vi "S4GUI_003.vi"(7 "Tab ObsEng":enum32{"Obs", "CCD modes", "Guider", "Eng"}(tab)) -> ()   [LabVIEW 2018] (continued)
                    n884 = property on="Read Mode 2" class="Ring (strict)"("Blinking"=w1549) -> ()  [unwired: 2 in, 2 out]
                    n885 = property on="Pre-amplification Gain 2" class="Ring (strict)"("Blinking"=w1551) -> ()  [unwired: 2 in, 2 out]
                  }
                }
                n886 = local read "Cameras Cluster"() -> (w1515:T7)
                n887 = Bundle By Name(cluster=w1515, "Current Configuration.Image Initial Line 2"=w1478, "Current Configuration.Image Initial Column 2"=w1476, "Current Configuration.Image Final Line 2"=w1479, "Current Configuration.Image FInal Column 2"=w1477, "Current Configuration.Vertical Binning 2"=w1482, "Current Configuration.Horizontal Binning 2"=w1513, "Current Configuration.Pre-amplification Gain 2"=w1481, "Current Configuration.CCD EM Gain 2"=w1480, "Current Configuration.Readout Rate 2"=w1475, "Current Configuration.Shutter Openning Time 2"=w1512, "Current Configuration.Shutter Closing Time 2"=w1511, "Current Configuration.Vertical Shift Speed 2"=w1510, "Current Configuration.Read Mode 2"=w1509, "Current Configuration.Vertical Clock Voltage 2"=w1508, "Current Configuration.A/D Channel 2"=w1507, "Current Configuration.Shutter Mode 2"=w1504, "Current Configuration.Shutter TTL 2"=w1505, "Current Configuration.Trigger Mode 2"=w1483, "Current Configuration.Frame Transfer 2"=w1484, "Current Configuration.Acquisition Mode 2"=w1506, "Current Configuration.CCD EM Mode 2"=w1474) -> (w1514:T7)
                n888 = local write "PA2"(w1469) -> ()
                n889 = local write "B2"(w1468) -> ()
                n890 = local write "EA2"(w1470) -> ()
                n891 = local write "SI2"(w1465) -> ()
                n892 = local write "RO2"(w1466) -> ()
                n893 = local write "G2"(w1467) -> ()
                n894 = local write "Cameras Cluster"(w1514) -> ()
                n895 = Compound Arithmetic op=AND(w1489, w1488, w1487, w1486, w1462, w1461, w1485, w1496, w1495, w1494, w1493, w1492, w1491, w1490, w1503, w1502, w1501, w1500, w1499, w1498, w1497) -> (w1460:bool)
                "CCD checked 2" <- w1460
                n896 = disable-structure shown="Disabled" {
                  disable-tunnel: w1460 -> [w1517 _]
                  frame Disabled {
                    n897 = Select(t=u32 1244955, s=w1517, f=u32 16718848) -> (s? t:f=w1520:u32)
                    n898 = property on="CCD checked 2" class="Bool (strict)"("Caption.BG Color"=w1520) -> ()  [unwired: 2 in, 2 out]
                  }
                  frame Enabled {
                  }
                }
                n899 = property on="Acquisition Mode 2" class="Ring (strict)"("DisabledEnum"=w1463) -> ()  [unwired: 2 in, 2 out]
                n900 = property on="Readout Rate 2" class="Ring (strict)"("DisabledEnum"=w1463) -> ()  [unwired: 2 in, 2 out]
                n901 = property on="Vertical Shift Speed 2" class="Ring (strict)"("DisabledEnum"=w1463) -> ()  [unwired: 2 in, 2 out]
                n902 = property on="CCD EM Mode 2" class="Ring (strict)"("DisabledEnum"=w1463) -> ()  [unwired: 2 in, 2 out]
                n903 = property on="Shutter Openning Time 2" class="DigNum (strict)"("DisabledEnum"=w1463) -> ()  [unwired: 2 in, 2 out]
                n904 = property on="Shutter Closing Time 2" class="DigNum (strict)"("DisabledEnum"=w1463) -> ()  [unwired: 2 in, 2 out]
                n905 = property on="Vertical Binning 2" class="DigNum (strict)"("DisabledEnum"=w1463) -> ()  [unwired: 2 in, 2 out]
                n906 = property on="Horizontal Binning 2" class="DigNum (strict)"("DisabledEnum"=w1463) -> ()  [unwired: 2 in, 2 out]
                n907 = property on="Trigger Mode 2" class="Ring (strict)"("DisabledEnum"=w1463) -> ()  [unwired: 2 in, 2 out]
                n908 = property on="Read Mode 2" class="Ring (strict)"("DisabledEnum"=w1463) -> ()  [unwired: 2 in, 2 out]
                n909 = property on="Pre-amplification Gain 2" class="Ring (strict)"("DisabledEnum"=w1463) -> ()  [unwired: 2 in, 2 out]
                n910 = property on="CCD EM Gain 2" class="DigNum (strict)"("DisabledEnum"=w1463) -> ()  [unwired: 2 in, 2 out]
                n911 = property on="Shutter Mode 2" class="Ring (strict)"("DisabledEnum"=w1463) -> ()  [unwired: 2 in, 2 out]
                n912 = property on="Shutter TTL 2" class="Ring (strict)"("DisabledEnum"=w1463) -> ()  [unwired: 2 in, 2 out]
                n913 = property on="Image FInal Column 2" class="DigNum (strict)"("DisabledEnum"=w1463) -> ()  [unwired: 2 in, 2 out]
                n914 = property on="Frame Transfer 2" class="Bool (strict)"("DisabledEnum"=w1463) -> ()  [unwired: 2 in, 2 out]
                n915 = property on="Vertical Clock Voltage 2" class="Ring (strict)"("DisabledEnum"=w1463) -> ()  [unwired: 2 in, 2 out]
                n916 = property on="A/D Channel 2" class="DigNum (strict)"("DisabledEnum"=w1463) -> ()  [unwired: 2 in, 2 out]
                n917 = property on="Image Initial Line 2" class="DigNum (strict)"("DisabledEnum"=w1463) -> ()  [unwired: 2 in, 2 out]
                n918 = property on="Image Initial Column 2" class="DigNum (strict)"("DisabledEnum"=w1463) -> ()  [unwired: 2 in, 2 out]
                n919 = property on="Image Final Line 2" class="DigNum (strict)"("DisabledEnum"=w1463) -> ()  [unwired: 2 in, 2 out]
              }
              frame #17 {
                # "Carrega coluna do Channel 3"
                # "Aba:  Eng->Camera"
                n920 = Unbundle By Name(w1679) -> ("ChannelC_CCD"=w1649:T29, "CHC_Checked Params"=w1664:T14, "ChannelC_Status.connection"=w1642:bool)
                n921 = Unbundle By Name(w1664) -> ("ACQUISITION_MODE"=w1631:bool, "TRIGGER_MODE"=w1630:bool, "READ_MODE"=w1629:bool, "PREAMP"=w1628:bool, "READOUT_RATE"=w1627:bool, "VERTICAL_SHIFT_SPEED"=w1626:bool, "EM_MODE"=w1625:bool, "EM_GAIN"=w1662:bool, "SHUTTER_MODE"=w1661:bool, "SHUTTER_TTL"=w1660:bool, "SHUTTER_OPENING_TIME"=w1659:bool, "SHUTTER_CLOSING_TIME"=w1641:bool, "VBIN"=w1633:bool, "HBIN"=w1632:bool, "INITIAL_LINE"=w1640:bool, "INITIAL_COLUMN"=w1639:bool, "FINAL_LINE"=w1638:bool, "FINAL_COLUMN"=w1637:bool, "FRAME_TRANSFER"=w1636:bool, "VERTICAL_CLOCK_VOLTAGE"=w1635:bool, "AD_CHANNEL"=w1634:bool)
                n922 = case shown="True" w1642 {
                  tunnel: w1649 -> [_ w1732]
                  tunnel: [w1725 w1731] -> w1648
                  tunnel: [w1725 w1730] -> w1647
                  tunnel: [w1725 w1729] -> w1646
                  tunnel: [w1725 w1728] -> w1645
                  tunnel: [w1725 w1727] -> w1644
                  tunnel: [w1725 w1726] -> w1643
                  frame False {
                    w1725 = ""
                  }
                  frame True {
                    n923 = stacked-sequence "Atualizacao dos indicadores inferiores do CANAL C da tela principal" {
                      tunnel: w1732 -> [w1747 w1750 w1755 w1764 w1767 w1771]
                      tunnel: [w1733 _ _ _ _ _] -> w1731
                      tunnel: [_ w1748 _ _ _ _] -> w1730
                      tunnel: [_ _ w1753 _ _ _] -> w1729
                      tunnel: [_ _ _ w1758 _ _] -> w1728
                      tunnel: [_ _ _ _ w1765 _] -> w1727
                      tunnel: [_ _ _ _ _ w1768] -> w1726
                      frame #0 {
                        # "SubImage"
                        n924 = Unbundle By Name(w1747) -> ("INITIAL_LINE"=w1745:u16, "FINAL_LINE"=w1744:u16, "INITIAL_COLUMN"=w1743:u16, "FINAL_COLUMN"=w1742:u16)
                        n925 = Number To Decimal String(number=w1745) -> (decimal integer string=w1741:string)  [unwired: 1 in]
                        n926 = Number To Decimal String(number=w1744) -> (decimal integer string=w1739:string)  [unwired: 1 in]
                        n927 = Number To Decimal String(number=w1743) -> (decimal integer string=w1737:string)  [unwired: 1 in]
                        n928 = Number To Decimal String(number=w1742) -> (decimal integer string=w1735:string)  [unwired: 1 in]
                        n929 = Concatenate Strings("[", w1741, ":", w1739, ",", w1737, ":", w1735, "]") -> (w1733:string)
                      }
                      frame #1 {
                        # "Em Active"
                        n930 = Unbundle By Name(w1750) -> ("EM_MODE"=w1749:u8)
                        n931 = case shown="0, Default" w1749 {
                          tunnel: ["Electron M." ("EmActive1") "Convent." ("EmActive1")] -> w1748
                          frame 0, Default {
                          }
                          frame 1 {
                          }
                        }
                      }
                      frame #2 {
                        # "Pre Amp"
                        n932 = Unbundle By Name(w1755) -> ("PREAMP"=w1754:u8)
                        n933 = case shown="1" w1754 {
                          tunnel: ["Gain 1" ("EmActive1") "Gain 2" ("EmActive1")] -> w1753
                          frame 0, Default {
                          }
                          frame 1 {
                          }
                        }
                      }
                      frame #3 {
                        # "Binning"
                        n934 = Unbundle By Name(w1764) -> ("VBIN"=w1763:u16, "HBIN"=w1762:u16)
                        n935 = Number To Decimal String(number=w1762) -> (decimal integer string=w1759:string)  [unwired: 1 in]
                        n936 = Number To Decimal String(number=w1763) -> (decimal integer string=w1761:string)  [unwired: 1 in]
                        n937 = Concatenate Strings(w1761, "x", w1759) -> (w1758:string)
                      }
                      frame #4 {
                        # "Gain"
                        n938 = Unbundle By Name(w1767) -> ("EM_GAIN"=w1766:u16)
                        n939 = Number To Decimal String(number=w1766) -> (decimal integer string=w1765:string)  [unwired: 1 in]
                      }
                      frame #5 {
                        # "Readout"
                        n940 = Unbundle By Name(w1771) -> ("EM_MODE"=w1770:u8, "READOUT_RATE"=w1769:u8)
                        n941 = case shown="0, Default" w1770 {
                          tunnel: w1769 -> [w1773 w1779]
                          tunnel: [w1772 w1778] -> w1768
                          frame 0, Default {
                            n942 = case shown="3" w1773 {
                              tunnel: ["30 MHz" ("EmActive1") "20 MHz" ("EmActive1") "10 MHz" ("EmActive1") "1 MHz" ("EmActive1")] -> w1772
                              frame 0, Default {
                              }
                              frame 1 {
                              }
                              frame 2 {
                              }
                              frame 3 {
                              }
                            }
                          }
                          frame 1 {
                            n943 = case shown="1" w1779 {
                              tunnel: ["1 MHz" ("EmActive1") "0.1 MHz" ("EmActive1")] -> w1778
                              frame 0, Default {
                              }
                              frame 1 {
                              }
                            }
                          }
                        }
                      }
                    }
                  }
                }
                n944 = Unbundle By Name(w1649) -> ("INITIAL_LINE"=w1654:u16, "INITIAL_COLUMN"=w1652:u16, "FINAL_LINE"=w1655:u16, "FINAL_COLUMN"=w1653:u16, "VBIN"=w1658:u16, "HBIN"=w1676:u16, "PREAMP"=w1657:u8, "EM_GAIN"=w1656:u16, "READOUT_RATE"=w1651:u8, "SHUTTER_OPENNING_TIME"=w1675:u16, "SHUTTER_CLOSING_TIME"=w1674:u16, "VERTICAL_SHIFT_SPEED"=w1673:u8, "READ_MODE"=w1672:u8, "VERTICAL_CLOCK_VOLTAGE"=w1671:u8, "AD_CHANNEL"=w1670:u32, "SHUTTER_MODE"=w1665:u8, "SHUTTER_TTL"=w1666:u8, "TRIGGER_MODE"=w1667:u8, "FRAME_TRANSFER"=w1668:bool, "ACQUISITION_MODE"=w1669:u8, "EM_MODE"=w1650:u8)
                n945 = local read "CH3 on"() -> (w1624:bool)
                n946 = case shown="True" w1624 {
                  tunnel: w1662 -> [_ w1705]
                  tunnel: w1661 -> [_ w1704]
                  tunnel: w1660 -> [_ w1702]
                  tunnel: w1659 -> [_ w1701]
                  tunnel: w1641 -> [_ w1700]
                  tunnel: w1640 -> [_ w1699]
                  tunnel: w1639 -> [_ w1698]
                  tunnel: w1638 -> [_ w1697]
                  tunnel: w1637 -> [_ w1696]
                  tunnel: w1636 -> [_ w1695]
                  tunnel: w1635 -> [_ w1694]
                  tunnel: w1634 -> [_ w1693]
                  tunnel: w1633 -> [_ w1692]
                  tunnel: w1632 -> [_ w1691]
                  tunnel: w1631 -> [_ w1690]
                  tunnel: w1630 -> [_ w1689]
                  tunnel: w1629 -> [_ w1688]
                  tunnel: w1628 -> [_ w1687]
                  tunnel: w1627 -> [_ w1686]
                  tunnel: w1626 -> [_ w1685]
                  tunnel: w1625 -> [_ w1684]
                  tunnel: [T12."Disabled and Grayed Out" ("Disabled") T12."Enabled" ("Disabled")] -> w1623
                  frame False {
                    w1680 = FALSE
                    n947 = property on="Image Initial Line 3" class="DigNum (strict)"("Blinking"=w1680) -> ()  [unwired: 2 in, 2 out]
                    n948 = property on="Image Initial Column 3" class="DigNum (strict)"("Blinking"=w1680) -> ()  [unwired: 2 in, 2 out]
                    n949 = property on="Image Final Line 3" class="DigNum (strict)"("Blinking"=w1680) -> ()  [unwired: 2 in, 2 out]
                    n950 = property on="Image FInal Column 3" class="DigNum (strict)"("Blinking"=w1680) -> ()  [unwired: 2 in, 2 out]
                    n951 = property on="Frame Transfer 3" class="Bool (strict)"("Blinking"=w1680) -> ()  [unwired: 2 in, 2 out]
                    n952 = property on="Vertical Clock Voltage 3" class="Ring (strict)"("Blinking"=w1680) -> ()  [unwired: 2 in, 2 out]
                    n953 = property on="A/D Channel 3" class="DigNum (strict)"("Blinking"=w1680) -> ()  [unwired: 2 in, 2 out]
                    n954 = property on="CCD EM Gain 3" class="DigNum (strict)"("Blinking"=w1680) -> ()  [unwired: 2 in, 2 out]
                    n955 = property on="Shutter Mode 3" class="Ring (strict)"("Blinking"=w1680) -> ()  [unwired: 2 in, 2 out]
                    n956 = property on="Shutter TTL 3" class="Ring (strict)"("Blinking"=w1680) -> ()  [unwired: 2 in, 2 out]
                    n957 = property on="Shutter Openning Time 3" class="DigNum (strict)"("Blinking"=w1680) -> ()  [unwired: 2 in, 2 out]
                    n958 = property on="Shutter Closing Time 3" class="DigNum (strict)"("Blinking"=w1680) -> ()  [unwired: 2 in, 2 out]
                    n959 = property on="Vertical Binning 3" class="DigNum (strict)"("Blinking"=w1680) -> ()  [unwired: 2 in, 2 out]
                    n960 = property on="Horizontal Binning 3" class="DigNum (strict)"("Blinking"=w1680) -> ()  [unwired: 2 in, 2 out]
                    n961 = property on="Acquisition Mode 3" class="Ring (strict)"("Blinking"=w1680) -> ()  [unwired: 2 in, 2 out]
                    n962 = property on="Vertical Shift Speed 3" class="Ring (strict)"("Blinking"=w1680) -> ()  [unwired: 2 in, 2 out]
                    n963 = property on="Trigger Mode 3" class="Ring (strict)"("Blinking"=w1680) -> ()  [unwired: 2 in, 2 out]
                    n964 = property on="Read Mode 3" class="Ring (strict)"("Blinking"=w1680) -> ()  [unwired: 2 in, 2 out]
                    n965 = property on="Readout Rate 3" class="Ring (strict)"("Blinking"=w1680) -> ()  [unwired: 2 in, 2 out]
                    n966 = property on="CCD EM Mode 3" class="Ring (strict)"("Blinking"=w1680) -> ()  [unwired: 2 in, 2 out]
                    n967 = property on="Pre-amplification Gain 3" class="Ring (strict)"("Blinking"=w1680) -> ()  [unwired: 2 in, 2 out]
                  }
                  frame True {
                    n968 = Not(x=w1699) -> (.not. x?=w1682:bool)
                    n969 = Not(x=w1698) -> (.not. x?=w1723:bool)
                    n970 = Not(x=w1697) -> (.not. x?=w1724:bool)
                    n971 = Not(x=w1696) -> (.not. x?=w1722:bool)
                    n972 = Not(x=w1695) -> (.not. x?=w1720:bool)
                    n973 = Not(x=w1694) -> (.not. x?=w1721:bool)
                    n974 = Not(x=w1693) -> (.not. x?=w1719:bool)
                    n975 = property on="Image FInal Column 3" class="DigNum (strict)"("Blinking"=w1722) -> ()  [unwired: 2 in, 2 out]
                    n976 = property on="Frame Transfer 3" class="Bool (strict)"("Blinking"=w1720) -> ()  [unwired: 2 in, 2 out]
                    n977 = property on="Vertical Clock Voltage 3" class="Ring (strict)"("Blinking"=w1721) -> ()  [unwired: 2 in, 2 out]
                    n978 = property on="Image Initial Line 3" class="DigNum (strict)"("Blinking"=w1682) -> ()  [unwired: 2 in, 2 out]
                    n979 = property on="Image Initial Column 3" class="DigNum (strict)"("Blinking"=w1723) -> ()  [unwired: 2 in, 2 out]
                    n980 = property on="Image Final Line 3" class="DigNum (strict)"("Blinking"=w1724) -> ()  [unwired: 2 in, 2 out]
                    n981 = property on="A/D Channel 3" class="DigNum (strict)"("Blinking"=w1719) -> ()  [unwired: 2 in, 2 out]
                    n982 = Not(x=w1701) -> (.not. x?=w1715:bool)
                    n983 = Not(x=w1700) -> (.not. x?=w1717:bool)
                    n984 = Not(x=w1692) -> (.not. x?=w1716:bool)
                    n985 = Not(x=w1691) -> (.not. x?=w1718:bool)
                    n986 = Not(x=w1705) -> (.not. x?=w1714:bool)
                    n987 = Not(x=w1704) -> (.not. x?=w1703:bool)
                    n988 = Not(x=w1702) -> (.not. x?=w1713:bool)
                    n989 = property on="Shutter Openning Time 3" class="DigNum (strict)"("Blinking"=w1715) -> ()  [unwired: 2 in, 2 out]
                    n990 = property on="Shutter Closing Time 3" class="DigNum (strict)"("Blinking"=w1717) -> ()  [unwired: 2 in, 2 out]
                    n991 = property on="Vertical Binning 3" class="DigNum (strict)"("Blinking"=w1716) -> ()  [unwired: 2 in, 2 out]
                    n992 = property on="Horizontal Binning 3" class="DigNum (strict)"("Blinking"=w1718) -> ()  [unwired: 2 in, 2 out]
                    n993 = property on="CCD EM Gain 3" class="DigNum (strict)"("Blinking"=w1714) -> ()  [unwired: 2 in, 2 out]
                    n994 = property on="Shutter Mode 3" class="Ring (strict)"("Blinking"=w1703) -> ()  [unwired: 2 in, 2 out]
                    n995 = property on="Shutter TTL 3" class="Ring (strict)"("Blinking"=w1713) -> ()  [unwired: 2 in, 2 out]
                    n996 = Not(x=w1690) -> (.not. x?=w1706:bool)
                    n997 = Not(x=w1686) -> (.not. x?=w1709:bool)
                    n998 = Not(x=w1685) -> (.not. x?=w1707:bool)
                    n999 = Not(x=w1684) -> (.not. x?=w1708:bool)
                    n1000 = Not(x=w1689) -> (.not. x?=w1711:bool)
                    n1001 = Not(x=w1688) -> (.not. x?=w1710:bool)
                    n1002 = Not(x=w1687) -> (.not. x?=w1712:bool)
                    n1003 = property on="Acquisition Mode 3" class="Ring (strict)"("Blinking"=w1706) -> ()  [unwired: 2 in, 2 out]
                    n1004 = property on="Readout Rate 3" class="Ring (strict)"("Blinking"=w1709) -> ()  [unwired: 2 in, 2 out]
                    n1005 = property on="Vertical Shift Speed 3" class="Ring (strict)"("Blinking"=w1707) -> ()  [unwired: 2 in, 2 out]
                    n1006 = property on="CCD EM Mode 3" class="Ring (strict)"("Blinking"=w1708) -> ()  [unwired: 2 in, 2 out]
                    n1007 = property on="Trigger Mode 3" class="Ring (strict)"("Blinking"=w1711) -> ()  [unwired: 2 in, 2 out]
                    n1008 = property on="Read Mode 3" class="Ring (strict)"("Blinking"=w1710) -> ()  [unwired: 2 in, 2 out]
                    n1009 = property on="Pre-amplification Gain 3" class="Ring (strict)"("Blinking"=w1712) -> ()  [unwired: 2 in, 2 out]
                  }
                }
                n1010 = local write "RO3"(w1643) -> ()
                n1011 = local write "B3"(w1645) -> ()
                n1012 = local write "PA3"(w1646) -> ()
                n1013 = local write "EA3"(w1647) -> ()
                n1014 = local write "G3"(w1644) -> ()
                n1015 = local write "SI3"(w1648) -> ()
                n1016 = local read "Cameras Cluster"() -> (w1678:T7)
                n1017 = Bundle By Name(cluster=w1678, "Current Configuration.Image Initial Line 3"=w1654, "Current Configuration.Image Initial Column 3"=w1652, "Current Configuration.Image Final Line 3"=w1655, "Current Configuration.Image FInal Column 3"=w1653, "Current Configuration.Vertical Binning 3"=w1658, "Current Configuration.Horizontal Binning 3"=w1676, "Current Configuration.Pre-amplification Gain 3"=w1657, "Current Configuration.CCD EM Gain 3"=w1656, "Current Configuration.Readout Rate 3"=w1651, "Current Configuration.Shutter Openning Time 3"=w1675, "Current Configuration.Shutter Closing Time 3"=w1674, "Current Configuration.Vertical Shift Speed 3"=w1673, "Current Configuration.Read Mode 3"=w1672, "Current Configuration.Vertical Clock Voltage 3"=w1671, "Current Configuration.A/D Channel 3"=w1670, "Current Configuration.Shutter Mode 3"=w1665, "Current Configuration.Shutter TTL 3"=w1666, "Current Configuration.Trigger Mode 3"=w1667, "Current Configuration.Frame Transfer 3"=w1668, "Current Configuration.Acquisition Mode 3"=w1669, "Current Configuration.CCD EM Mode 3"=w1650) -> (w1677:T7)
                n1018 = local write "Cameras Cluster"(w1677) -> ()
                n1019 = Compound Arithmetic op=AND(w1631, w1630, w1629, w1628, w1627, w1626, w1625, w1662, w1661, w1660, w1659, w1641, w1633, w1632, w1640, w1639, w1638, w1637, w1636, w1635, w1634) -> (→"CCD checked 3":bool)
                n1020 = property on="Image Initial Line 3" class="DigNum (strict)"("DisabledEnum"=w1623) -> ()  [unwired: 2 in, 2 out]
                n1021 = property on="Image Initial Column 3" class="DigNum (strict)"("DisabledEnum"=w1623) -> ()  [unwired: 2 in, 2 out]
                n1022 = property on="Image Final Line 3" class="DigNum (strict)"("DisabledEnum"=w1623) -> ()  [unwired: 2 in, 2 out]
                n1023 = property on="Image FInal Column 3" class="DigNum (strict)"("DisabledEnum"=w1623) -> ()  [unwired: 2 in, 2 out]
                n1024 = property on="Frame Transfer 3" class="Bool (strict)"("DisabledEnum"=w1623) -> ()  [unwired: 2 in, 2 out]
                n1025 = property on="Horizontal Binning 3" class="DigNum (strict)"("DisabledEnum"=w1623) -> ()  [unwired: 2 in, 2 out]
                n1026 = property on="Vertical Clock Voltage 3" class="Ring (strict)"("DisabledEnum"=w1623) -> ()  [unwired: 2 in, 2 out]
                n1027 = property on="CCD EM Gain 3" class="DigNum (strict)"("DisabledEnum"=w1623) -> ()  [unwired: 2 in, 2 out]
                n1028 = property on="Shutter Mode 3" class="Ring (strict)"("DisabledEnum"=w1623) -> ()  [unwired: 2 in, 2 out]
                n1029 = property on="Shutter Openning Time 3" class="DigNum (strict)"("DisabledEnum"=w1623) -> ()  [unwired: 2 in, 2 out]
                n1030 = property on="Shutter Closing Time 3" class="DigNum (strict)"("DisabledEnum"=w1623) -> ()  [unwired: 2 in, 2 out]
                n1031 = property on="Vertical Binning 3" class="DigNum (strict)"("DisabledEnum"=w1623) -> ()  [unwired: 2 in, 2 out]
                n1032 = property on="Shutter TTL 3" class="Ring (strict)"("DisabledEnum"=w1623) -> ()  [unwired: 2 in, 2 out]
                n1033 = property on="Pre-amplification Gain 3" class="Ring (strict)"("DisabledEnum"=w1623) -> ()  [unwired: 2 in, 2 out]
                n1034 = property on="Acquisition Mode 3" class="Ring (strict)"("DisabledEnum"=w1623) -> ()  [unwired: 2 in, 2 out]
                n1035 = property on="Trigger Mode 3" class="Ring (strict)"("DisabledEnum"=w1623) -> ()  [unwired: 2 in, 2 out]
                n1036 = property on="Read Mode 3" class="Ring (strict)"("DisabledEnum"=w1623) -> ()  [unwired: 2 in, 2 out]
                n1037 = property on="Readout Rate 3" class="Ring (strict)"("DisabledEnum"=w1623) -> ()  [unwired: 2 in, 2 out]
                n1038 = property on="A/D Channel 3" class="DigNum (strict)"("DisabledEnum"=w1623) -> ()  [unwired: 2 in, 2 out]
                n1039 = property on="Vertical Shift Speed 3" class="Ring (strict)"("DisabledEnum"=w1623) -> ()  [unwired: 2 in, 2 out]
                n1040 = property on="CCD EM Mode 3" class="Ring (strict)"("DisabledEnum"=w1623) -> ()  [unwired: 2 in, 2 out]
              }
              frame #18 {
                # "Carrega coluna do Channel 4"
                # "Aba:  Eng->Camera"
                n1041 = Unbundle By Name(w1838) -> ("ChannelD_CCD"=w1791:T29, "CHD_Checked Params"=w1823:T14, "ChannelD_Status.connection"=w1790:bool)
                n1042 = Unbundle By Name(w1823) -> ("ACQUISITION_MODE"=w1807:bool, "TRIGGER_MODE"=w1806:bool, "READ_MODE"=w1805:bool, "PREAMP"=w1804:bool, "READOUT_RATE"=w1803:bool, "VERTICAL_SHIFT_SPEED"=w1802:bool, "EM_MODE"=w1801:bool, "EM_GAIN"=w1814:bool, "SHUTTER_MODE"=w1813:bool, "SHUTTER_TTL"=w1812:bool, "SHUTTER_OPENING_TIME"=w1811:bool, "SHUTTER_CLOSING_TIME"=w1810:bool, "VBIN"=w1809:bool, "HBIN"=w1808:bool, "INITIAL_LINE"=w1821:bool, "INITIAL_COLUMN"=w1820:bool, "FINAL_LINE"=w1819:bool, "FINAL_COLUMN"=w1818:bool, "FRAME_TRANSFER"=w1817:bool, "VERTICAL_CLOCK_VOLTAGE"=w1816:bool, "AD_CHANNEL"=w1815:bool)
                n1043 = case shown="True" w1790 {
                  tunnel: w1791 -> [_ w1891]
                  tunnel: [w1884 w1890] -> w1789
                  tunnel: [w1884 w1889] -> w1788
                  tunnel: [w1884 w1888] -> w1787
                  tunnel: [w1884 w1887] -> w1786
                  tunnel: [w1884 w1886] -> w1785
                  tunnel: [w1884 w1885] -> w1784
                  frame False {
                    w1884 = ""
                  }
                  frame True {
                    n1044 = stacked-sequence "Atualizacao dos indicadores inferiores do CANAL D da tela principal" {
                      tunnel: w1891 -> [w1906 w1909 w1914 w1923 w1926 w1930]
                      tunnel: [w1892 _ _ _ _ _] -> w1890
                      tunnel: [_ w1907 _ _ _ _] -> w1889
                      tunnel: [_ _ w1912 _ _ _] -> w1888
                      tunnel: [_ _ _ w1917 _ _] -> w1887
                      tunnel: [_ _ _ _ w1924 _] -> w1886
                      tunnel: [_ _ _ _ _ w1927] -> w1885
                      frame #0 {
                        # "SubImage"
                        n1045 = Unbundle By Name(w1906) -> ("INITIAL_LINE"=w1904:u16, "FINAL_LINE"=w1903:u16, "INITIAL_COLUMN"=w1902:u16, "FINAL_COLUMN"=w1901:u16)
                        n1046 = Number To Decimal String(number=w1904) -> (decimal integer string=w1900:string)  [unwired: 1 in]
                        n1047 = Number To Decimal String(number=w1903) -> (decimal integer string=w1898:string)  [unwired: 1 in]
                        n1048 = Number To Decimal String(number=w1902) -> (decimal integer string=w1896:string)  [unwired: 1 in]
                        n1049 = Number To Decimal String(number=w1901) -> (decimal integer string=w1894:string)  [unwired: 1 in]
                        n1050 = Concatenate Strings("[", w1900, ":", w1898, ",", w1896, ":", w1894, "]") -> (w1892:string)
                      }
                      frame #1 {
                        # "Em Active"
                        n1051 = Unbundle By Name(w1909) -> ("EM_MODE"=w1908:u8)
                        n1052 = case shown="0, Default" w1908 {
                          tunnel: ["Electron M." ("EmActive1") "Convent." ("EmActive1")] -> w1907
                          frame 0, Default {
                          }
                          frame 1 {
                          }
                        }
                      }
                      frame #2 {
                        # "Pre Amp"
                        n1053 = Unbundle By Name(w1914) -> ("PREAMP"=w1913:u8)
                        n1054 = case shown="1" w1913 {
                          tunnel: ["Gain 1" ("EmActive1") "Gain 2" ("EmActive1")] -> w1912
                          frame 0, Default {
                          }
                          frame 1 {
                          }
                        }
                      }
                      frame #3 {
                        # "Binning"
                        n1055 = Unbundle By Name(w1923) -> ("VBIN"=w1922:u16, "HBIN"=w1921:u16)
                        n1056 = Number To Decimal String(number=w1921) -> (decimal integer string=w1918:string)  [unwired: 1 in]
                        n1057 = Number To Decimal String(number=w1922) -> (decimal integer string=w1920:string)  [unwired: 1 in]
                        n1058 = Concatenate Strings(w1920, "x", w1918) -> (w1917:string)
                      }
                      frame #4 {
                        # "Gain"
                        n1059 = Unbundle By Name(w1926) -> ("EM_GAIN"=w1925:u16)
                        n1060 = Number To Decimal String(number=w1925) -> (decimal integer string=w1924:string)  [unwired: 1 in]
                      }
                      frame #5 {
                        # "Readout"
                        n1061 = Unbundle By Name(w1930) -> ("EM_MODE"=w1929:u8, "READOUT_RATE"=w1928:u8)
                        n1062 = case shown="0, Default" w1929 {
                          tunnel: w1928 -> [w1932 w1938]
                          tunnel: [w1931 w1937] -> w1927
                          frame 0, Default {
                            n1063 = case shown="3" w1932 {
                              tunnel: ["30 MHz" ("EmActive1") "20 MHz" ("EmActive1") "10 MHz" ("EmActive1") "1 MHz" ("EmActive1")] -> w1931
                              frame 0, Default {
                              }
                              frame 1 {
                              }
                              frame 2 {
                              }
                              frame 3 {
                              }
                            }
                          }
                          frame 1 {
                            n1064 = case shown="0, Default" w1938 {
                              tunnel: ["1 MHz" ("EmActive1") "0.1 MHz" ("EmActive1")] -> w1937
                              frame 0, Default {
                              }
                              frame 1 {
                              }
                            }
                          }
                        }
                      }
                    }
                  }
                }
                n1065 = Unbundle By Name(w1791) -> ("INITIAL_LINE"=w1796:u16, "INITIAL_COLUMN"=w1794:u16, "FINAL_LINE"=w1797:u16, "FINAL_COLUMN"=w1795:u16, "VBIN"=w1800:u16, "HBIN"=w1835:u16, "PREAMP"=w1799:u8, "EM_GAIN"=w1798:u16, "READOUT_RATE"=w1793:u8, "SHUTTER_OPENNING_TIME"=w1834:u16, "SHUTTER_CLOSING_TIME"=w1833:u16, "VERTICAL_SHIFT_SPEED"=w1832:u8, "READ_MODE"=w1831:u8, "VERTICAL_CLOCK_VOLTAGE"=w1830:u8, "AD_CHANNEL"=w1829:u32, "SHUTTER_MODE"=w1824:u8, "SHUTTER_TTL"=w1825:u8, "TRIGGER_MODE"=w1826:u8, "FRAME_TRANSFER"=w1827:bool, "ACQUISITION_MODE"=w1828:u8, "EM_MODE"=w1792:u8)
                n1066 = local read "CH4 on"() -> (w1783:bool)
                n1067 = case shown="False" w1783 {
                  tunnel: w1821 -> [_ w1863]
                  tunnel: w1820 -> [_ w1862]
                  tunnel: w1819 -> [_ w1861]
                  tunnel: w1818 -> [_ w1860]
                  tunnel: w1817 -> [_ w1859]
                  tunnel: w1816 -> [_ w1858]
                  tunnel: w1815 -> [_ w1857]
                  tunnel: w1814 -> [_ w1856]
                  tunnel: w1813 -> [_ w1855]
                  tunnel: w1812 -> [_ w1854]
                  tunnel: w1811 -> [_ w1853]
                  tunnel: w1810 -> [_ w1852]
                  tunnel: w1809 -> [_ w1851]
                  tunnel: w1808 -> [_ w1850]
                  tunnel: w1807 -> [_ w1849]
                  tunnel: w1806 -> [_ w1848]
                  tunnel: w1805 -> [_ w1847]
                  tunnel: w1804 -> [_ w1845]
                  tunnel: w1803 -> [_ w1844]
                  tunnel: w1802 -> [_ w1843]
                  tunnel: w1801 -> [_ w1842]
                  tunnel: [T12."Disabled and Grayed Out" ("Disabled") T12."Enabled" ("Disabled")] -> w1782
                  frame False {
                    w1840 = FALSE ("Blinking")
                    n1068 = property on="Image FInal Column 4" class="DigNum (strict)"("Blinking"=w1840) -> ()  [unwired: 2 in, 2 out]
                    n1069 = property on="Frame Transfer 4" class="Bool (strict)"("Blinking"=w1840) -> ()  [unwired: 2 in, 2 out]
                    n1070 = property on="Vertical Clock Voltage 4" class="Ring (strict)"("Blinking"=w1840) -> ()  [unwired: 2 in, 2 out]
                    n1071 = property on="A/D Channel 4" class="DigNum (strict)"("Blinking"=w1840) -> ()  [unwired: 2 in, 2 out]
                    n1072 = property on="Image Initial Line 4" class="DigNum (strict)"("Blinking"=w1840) -> ()  [unwired: 2 in, 2 out]
                    n1073 = property on="Image Initial Column 4" class="DigNum (strict)"("Blinking"=w1840) -> ()  [unwired: 2 in, 2 out]
                    n1074 = property on="Image Final Line 4" class="DigNum (strict)"("Blinking"=w1840) -> ()  [unwired: 2 in, 2 out]
                    n1075 = property on="Shutter Openning Time 4" class="DigNum (strict)"("Blinking"=w1840) -> ()  [unwired: 2 in, 2 out]
                    n1076 = property on="Shutter Closing Time 4" class="DigNum (strict)"("Blinking"=w1840) -> ()  [unwired: 2 in, 2 out]
                    n1077 = property on="Vertical Binning 4" class="DigNum (strict)"("Blinking"=w1840) -> ()  [unwired: 2 in, 2 out]
                    n1078 = property on="Horizontal Binning 4" class="DigNum (strict)"("Blinking"=w1840) -> ()  [unwired: 2 in, 2 out]
                    n1079 = property on="CCD EM Gain 4" class="DigNum (strict)"("Blinking"=w1840) -> ()  [unwired: 2 in, 2 out]
                    n1080 = property on="Shutter Mode 4" class="Ring (strict)"("Blinking"=w1840) -> ()  [unwired: 2 in, 2 out]
                    n1081 = property on="Shutter TTL 4" class="Ring (strict)"("Blinking"=w1840) -> ()  [unwired: 2 in, 2 out]
                    n1082 = property on="Acquisition Mode 4" class="Ring (strict)"("Blinking"=w1840) -> ()  [unwired: 2 in, 2 out]
                    n1083 = property on="Readout Rate 4" class="Ring (strict)"("Blinking"=w1840) -> ()  [unwired: 2 in, 2 out]
                    n1084 = property on="Vertical Shift Speed 4" class="Ring (strict)"("Blinking"=w1840) -> ()  [unwired: 2 in, 2 out]
                    n1085 = property on="CCD EM Mode 4" class="Ring (strict)"("Blinking"=w1840) -> ()  [unwired: 2 in, 2 out]
                    n1086 = property on="Trigger Mode 4" class="Ring (strict)"("Blinking"=w1840) -> ()  [unwired: 2 in, 2 out]
                    n1087 = property on="Read Mode 4" class="Ring (strict)"("Blinking"=w1840) -> ()  [unwired: 2 in, 2 out]
                    n1088 = property on="Pre-amplification Gain 4" class="Ring (strict)"("Blinking"=w1840) -> ()  [unwired: 2 in, 2 out]
                  }
                  frame True {
                    n1089 = Not(x=w1860) -> (.not. x?=w1880:bool)
                    n1090 = Not(x=w1859) -> (.not. x?=w1878:bool)
                    n1091 = Not(x=w1858) -> (.not. x?=w1879:bool)
                    n1092 = Not(x=w1857) -> (.not. x?=w1877:bool)
                    n1093 = Not(x=w1863) -> (.not. x?=w1882:bool)
                    n1094 = Not(x=w1862) -> (.not. x?=w1881:bool)
                    n1095 = Not(x=w1861) -> (.not. x?=w1883:bool)
                    n1096 = property on="Image FInal Column 4" class="DigNum (strict)"("Blinking"=w1880) -> ()  [unwired: 2 in, 2 out]
                    n1097 = property on="Frame Transfer 4" class="Bool (strict)"("Blinking"=w1878) -> ()  [unwired: 2 in, 2 out]
                    n1098 = property on="Vertical Clock Voltage 4" class="Ring (strict)"("Blinking"=w1879) -> ()  [unwired: 2 in, 2 out]
                    n1099 = property on="A/D Channel 4" class="DigNum (strict)"("Blinking"=w1877) -> ()  [unwired: 2 in, 2 out]
                    n1100 = property on="Image Initial Line 4" class="DigNum (strict)"("Blinking"=w1882) -> ()  [unwired: 2 in, 2 out]
                    n1101 = property on="Image Initial Column 4" class="DigNum (strict)"("Blinking"=w1881) -> ()  [unwired: 2 in, 2 out]
                    n1102 = property on="Image Final Line 4" class="DigNum (strict)"("Blinking"=w1883) -> ()  [unwired: 2 in, 2 out]
                    n1103 = Not(x=w1853) -> (.not. x?=w1873:bool)
                    n1104 = Not(x=w1852) -> (.not. x?=w1875:bool)
                    n1105 = Not(x=w1851) -> (.not. x?=w1874:bool)
                    n1106 = Not(x=w1850) -> (.not. x?=w1876:bool)
                    n1107 = Not(x=w1856) -> (.not. x?=w1871:bool)
                    n1108 = Not(x=w1855) -> (.not. x?=w1872:bool)
                    n1109 = Not(x=w1854) -> (.not. x?=w1870:bool)
                    n1110 = property on="Shutter Openning Time 4" class="DigNum (strict)"("Blinking"=w1873) -> ()  [unwired: 2 in, 2 out]
                    n1111 = property on="Shutter Closing Time 4" class="DigNum (strict)"("Blinking"=w1875) -> ()  [unwired: 2 in, 2 out]
                    n1112 = property on="Vertical Binning 4" class="DigNum (strict)"("Blinking"=w1874) -> ()  [unwired: 2 in, 2 out]
                    n1113 = property on="Horizontal Binning 4" class="DigNum (strict)"("Blinking"=w1876) -> ()  [unwired: 2 in, 2 out]
                    n1114 = property on="CCD EM Gain 4" class="DigNum (strict)"("Blinking"=w1871) -> ()  [unwired: 2 in, 2 out]
                    n1115 = property on="Shutter Mode 4" class="Ring (strict)"("Blinking"=w1872) -> ()  [unwired: 2 in, 2 out]
                    n1116 = property on="Shutter TTL 4" class="Ring (strict)"("Blinking"=w1870) -> ()  [unwired: 2 in, 2 out]
                    n1117 = Not(x=w1849) -> (.not. x?=w1864:bool)
                    n1118 = Not(x=w1844) -> (.not. x?=w1867:bool)
                    n1119 = Not(x=w1843) -> (.not. x?=w1865:bool)
                    n1120 = Not(x=w1842) -> (.not. x?=w1866:bool)
                    n1121 = Not(x=w1848) -> (.not. x?=w1868:bool)
                    n1122 = Not(x=w1847) -> (.not. x?=w1846:bool)
                    n1123 = Not(x=w1845) -> (.not. x?=w1869:bool)
                    n1124 = property on="Acquisition Mode 4" class="Ring (strict)"("Blinking"=w1864) -> ()  [unwired: 2 in, 2 out]
                    n1125 = property on="Readout Rate 4" class="Ring (strict)"("Blinking"=w1867) -> ()  [unwired: 2 in, 2 out]
                    n1126 = property on="Vertical Shift Speed 4" class="Ring (strict)"("Blinking"=w1865) -> ()  [unwired: 2 in, 2 out]
                    n1127 = property on="CCD EM Mode 4" class="Ring (strict)"("Blinking"=w1866) -> ()  [unwired: 2 in, 2 out]
                    n1128 = property on="Trigger Mode 4" class="Ring (strict)"("Blinking"=w1868) -> ()  [unwired: 2 in, 2 out]
                    n1129 = property on="Read Mode 4" class="Ring (strict)"("Blinking"=w1846) -> ()  [unwired: 2 in, 2 out]
                    n1130 = property on="Pre-amplification Gain 4" class="Ring (strict)"("Blinking"=w1869) -> ()  [unwired: 2 in, 2 out]
                  }
                }
                n1131 = local write "SI4"(w1789) -> ()
                n1132 = local write "RO4"(w1784) -> ()
                n1133 = local write "PA4"(w1787) -> ()
                n1134 = local write "EA4"(w1788) -> ()
                n1135 = local write "G4"(w1785) -> ()
                n1136 = local write "B4"(w1786) -> ()
                n1137 = local read "Cameras Cluster"() -> (w1837:T7)
                n1138 = Bundle By Name(cluster=w1837, "Current Configuration.Image Initial Line 4"=w1796, "Current Configuration.Image Initial Column 4"=w1794, "Current Configuration.Image Final Line 4"=w1797, "Current Configuration.Image FInal Column 4"=w1795, "Current Configuration.Vertical Binning 4"=w1800, "Current Configuration.Horizontal Binning 4"=w1835, "Current Configuration.Pre-amplification Gain 4"=w1799, "Current Configuration.CCD EM Gain 4"=w1798, "Current Configuration.Readout Rate 4"=w1793, "Current Configuration.Shutter Openning Time 4"=w1834, "Current Configuration.Shutter Closing Time 4"=w1833, "Current Configuration.Vertical Shift Speed 4"=w1832, "Current Configuration.Read Mode 4"=w1831, "Current Configuration.Vertical Clock Voltage 4"=w1830, "Current Configuration.A/D Channel 4"=w1829, "Current Configuration.Shutter Mode 4"=w1824, "Current Configuration.Shutter TTL 4"=w1825, "Current Configuration.Trigger Mode 4"=w1826, "Current Configuration.Frame Transfer 4"=w1827, "Current Configuration.Acquisition Mode 4"=w1828, "Current Configuration.CCD EM Mode 4"=w1792) -> (w1836:T7)
                n1139 = local write "Cameras Cluster"(w1836) -> ()
                n1140 = Compound Arithmetic op=AND(w1807, w1806, w1805, w1804, w1803, w1802, w1801, w1814, w1813, w1812, w1811, w1810, w1809, w1808, w1821, w1820, w1819, w1818, w1817, w1816, w1815) -> (→"CCD checked 4":bool)
                n1141 = property on="Image FInal Column 4" class="DigNum (strict)"("DisabledEnum"=w1782) -> ()  [unwired: 2 in, 2 out]
                n1142 = property on="Frame Transfer 4" class="Bool (strict)"("DisabledEnum"=w1782) -> ()  [unwired: 2 in, 2 out]
                n1143 = property on="Vertical Clock Voltage 4" class="Ring (strict)"("DisabledEnum"=w1782) -> ()  [unwired: 2 in, 2 out]
                n1144 = property on="A/D Channel 4" class="DigNum (strict)"("DisabledEnum"=w1782) -> ()  [unwired: 2 in, 2 out]
                n1145 = property on="Image Initial Line 4" class="DigNum (strict)"("DisabledEnum"=w1782) -> ()  [unwired: 2 in, 2 out]
                n1146 = property on="Image Initial Column 4" class="DigNum (strict)"("DisabledEnum"=w1782) -> ()  [unwired: 2 in, 2 out]
                n1147 = property on="Image Final Line 4" class="DigNum (strict)"("DisabledEnum"=w1782) -> ()  [unwired: 2 in, 2 out]
                n1148 = property on="Shutter Openning Time 4" class="DigNum (strict)"("DisabledEnum"=w1782) -> ()  [unwired: 2 in, 2 out]
                n1149 = property on="Shutter Closing Time 4" class="DigNum (strict)"("DisabledEnum"=w1782) -> ()  [unwired: 2 in, 2 out]
                n1150 = property on="Vertical Binning 4" class="DigNum (strict)"("DisabledEnum"=w1782) -> ()  [unwired: 2 in, 2 out]
                n1151 = property on="Horizontal Binning 4" class="DigNum (strict)"("DisabledEnum"=w1782) -> ()  [unwired: 2 in, 2 out]
                n1152 = property on="Acquisition Mode 4" class="Ring (strict)"("DisabledEnum"=w1782) -> ()  [unwired: 2 in, 2 out]
                n1153 = property on="CCD EM Gain 4" class="DigNum (strict)"("DisabledEnum"=w1782) -> ()  [unwired: 2 in, 2 out]
                n1154 = property on="Shutter Mode 4" class="Ring (strict)"("DisabledEnum"=w1782) -> ()  [unwired: 2 in, 2 out]
                n1155 = property on="Shutter TTL 4" class="Ring (strict)"("DisabledEnum"=w1782) -> ()  [unwired: 2 in, 2 out]
                n1156 = property on="Readout Rate 4" class="Ring (strict)"("DisabledEnum"=w1782) -> ()  [unwired: 2 in, 2 out]
                n1157 = property on="Vertical Shift Speed 4" class="Ring (strict)"("DisabledEnum"=w1782) -> ()  [unwired: 2 in, 2 out]
                n1158 = property on="CCD EM Mode 4" class="Ring (strict)"("DisabledEnum"=w1782) -> ()  [unwired: 2 in, 2 out]
                n1159 = property on="Trigger Mode 4" class="Ring (strict)"("DisabledEnum"=w1782) -> ()  [unwired: 2 in, 2 out]
                n1160 = property on="Read Mode 4" class="Ring (strict)"("DisabledEnum"=w1782) -> ()  [unwired: 2 in, 2 out]
                n1161 = property on="Pre-amplification Gain 4" class="Ring (strict)"("DisabledEnum"=w1782) -> ()  [unwired: 2 in, 2 out]
              }
              frame #19 {
                n1162 = Unbundle By Name(w1948) -> ("object_suffix"=w1947:string, "dflat_suffix"=w1946:string, "sflat_suffix"=w1945:string, "dark_suffix"=w1944:string, "zero_suffix"=w1943:string, "focus_suffix"=w1942:string, "suffixAlertVisible"=w1941:bool)
                n1163 = local write "object suffix"(w1947) -> ()
                n1164 = local write "dflat suffix"(w1946) -> ()
                n1165 = local write "sflat suffix"(w1945) -> ()
                n1166 = local write "dark suffix"(w1944) -> ()
                n1167 = local write "zero suffix"(w1943) -> ()
                n1168 = local write "focus suffix"(w1942) -> ()
                n1169 = property on="suffix alert" class="Str"("Visible"=w1941) -> ()  [unwired: 2 in, 2 out]
                n1170 = case shown="True" w1951 {
                  tunnel: [w1952 w1988] -> w1949
                  tunnel: [w1952 w1972] -> w1950
                  tunnel: w1948 -> [_ w1978]
                  frame False {
                    w1952 = FALSE
                  }
                  frame True {
                    w1958 = TRUE
                    # "Pelo menos 1 canal deve \nestar habilitado"
                    n1171 = local read "Preview Temp."() -> (w1977:dbl)
                    n1172 = Unbundle By Name(w1978) -> ("ChannelA_Status.target  temp"=w1974:i16, "ChannelB_Status.target  temp"=w1976:i16, "ChannelC_Status.target  temp"=w1975:i16, "ChannelD_Status.target  temp"=w1973:i16)
                    n1173 = property on="CCD checked 3" class="Bool (strict)"() -> ("Value"=w1984:bool)  [unwired: 2 in, 2 out]
                    n1174 = local read "CH3 on"() -> (w1968:bool)
                    n1175 = local read "CH1on"() -> (w1970:bool)
                    n1176 = property on="CCD checked 2" class="Bool (strict)"() -> ("Value"=w1987:bool)  [unwired: 2 in, 2 out]
                    n1177 = local read "CH2on"() -> (w1969:bool)
                    n1178 = property on="CCD checked 1" class="Bool (strict)"() -> ("Value"=w1991:bool)  [unwired: 2 in, 2 out]
                    n1179 = property on="CCD checked 4" class="Bool (strict)"() -> ("Value"=w1981:bool)  [unwired: 2 in, 2 out]
                    n1180 = local read "CH4 on"() -> (w1967:bool)
                    n1181 = To Word Integer(number=w1977) -> (16bit integer=w1971:i16)
                    n1182 = Select(t=w1991, s=w1970, f=TRUE) -> (s? t:f=w1989:bool)
                    n1183 = local read "CH3 on"() -> (w1960:bool)
                    n1184 = local read "CH4 on"() -> (w1959:bool)
                    n1185 = Compound Arithmetic op=OR(w1970, w1969, w1968, w1967) -> (w1957:bool)
                    n1186 = local read "CH2on"() -> (w1961:bool)
                    n1187 = Select(t=w1984, s=w1968, f=TRUE) -> (s? t:f=w1982:bool)
                    n1188 = Select(t=w1987, s=w1969, f=TRUE) -> (s? t:f=w1985:bool)
                    n1189 = Select(t=w1981, s=w1967, f=TRUE) -> (s? t:f=w1979:bool)
                    n1190 = Equal?(x=w1971, y=w1976) -> (x = y?=w1965:bool)
                    n1191 = Equal?(x=w1971, y=w1975) -> (x = y?=w1964:bool)
                    n1192 = Equal?(x=w1971, y=w1973) -> (x = y?=w1963:bool)
                    n1193 = Equal?(x=w1971, y=w1974) -> (x = y?=w1966:bool)
                    n1194 = local read "CH1on"() -> (w1962:bool)
                    n1195 = Select(t=w1966, s=w1962, f=w1958) -> (s? t:f=w1956:bool)
                    n1196 = Select(t=w1964, s=w1960, f=w1958) -> (s? t:f=w1954:bool)
                    n1197 = Select(t=w1963, s=w1959, f=w1958) -> (s? t:f=w1953:bool)
                    n1198 = Select(t=w1965, s=w1961, f=w1958) -> (s? t:f=w1955:bool)
                    n1199 = Compound Arithmetic op=AND(w1989, w1985, w1982, w1979, w1957) -> (w1988:bool)
                    n1200 = Compound Arithmetic op=AND(w1957, w1956, w1955, w1954, w1953) -> (w1972:bool)
                  }
                }
                "SET Temp status" <- w1950
                "SET CCD status" <- w1949
              }
            }
            n1201 = call-dynamic "Read Obs_state.vi"("error in (no error)"=w335, "S4ACS_GUI in"=w336) -> ("error out"=w312:errorcluster, "Obs_state"=w332:u32, "S4ACS_GUI out"=w313:refnum<class "S4GUI.lvclass">)  [unwired: 7 in]
            n1202 = In Range and Coerce(upper limit=u32 226, x=w332, lower limit=u32 220 ("upper limit")) -> (In Range?=w330:bool)  [unwired: 1 out]
            n1203 = call-dynamic "Read TelFocus.lvclass.vi"("error in (no error)"=w312, "S4GUI in"=w313) -> ("error out"=w310:errorcluster, "TelFocus.lvclass"=w311:refnum<class "TelFocus.lvclass">)  [unwired: 7 in, 1 out]
            n1204 = Select(t="STOP", s=w330, f="INIT") -> (s? t:f=w329:string)
            n1205 = call-dynamic "Read focus #stepsdone.vi"("error in (no error)"=w310, "TelFocus in"=w311) -> ("focus #stepsdone"=→"steps done":u32)  [unwired: 7 in, 2 out]
            n1206 = property on="Init mode" class="Bool"(error in=w312, "Blinking"=w330, "Caption.Visible"=w330, "BoolText.Text"=w329) -> (error out=w331:errorcluster)  [unwired: 1 in, 1 out]
            n1207 = call-dynamic "Read cyclesDone.vi"("error in (no error)"=w331, "S4GUI in"=w313) -> ("error out"=w323:errorcluster, "cyclesDone"=w315:u32, "S4GUI out"=w325:refnum<class "S4GUI.lvclass">)  [unwired: 7 in]
            "#Cycles Done" <- w315
            n1208 = call-dynamic "Read cycles wprot.vi"("error in (no error)"=w323, "S4GUI in"=w325) -> ("cycles wprot"=→"Cycles Counter":u32)  [unwired: 7 in, 2 out]
            n1209 = Number To Decimal String(number=w315) -> (decimal integer string=w316:string)  [unwired: 1 in]
            n1210 = Concatenate Strings("#Cycles Done ", w316) -> (w314:string)
            n1211 = property on="#Cycles Done" class="Slide (strict)"("Caption.Text"=w314) -> ()  [unwired: 2 in, 2 out]
            n1212 = call "Read Instrument.lvclass.vi"("error in (no error)"=w323, "S4ACS_GUI in"=w325) -> ("error out"=w340:errorcluster, "Instrument.lvclass"=w338:refnum<class "Instrument.lvclass">, "S4ACS_GUI out"=w341:refnum<class "S4GUI.lvclass">)  [unwired: 7 in]
            n1213 = call-dynamic "Write mode.vi"("error in (no error)"=w340, "mode"=w326, "Instrument in"=w338) -> ("error out"=w339:errorcluster, "Instrument out"=w337:refnum<class "Instrument.lvclass">)  [unwired: 7 in]
            n1214 = call "Write Instrument.lvclass.vi"("error in (no error)"=w339, "Instrument.lvclass"=w337, "S4ACS_GUI in"=w341) -> ("error out"=w321:errorcluster, "S4ACS_GUI out"=w322:refnum<class "S4GUI.lvclass">)  [unwired: 7 in]
            n1215 = call-dynamic "Read Error Msg.vi"("error in (no error)"=w321, "S4GUI in"=w322) -> ("error out"=w318:errorcluster, "Error Msg"=w300:string, "S4GUI out"=w305:refnum<class "S4GUI.lvclass">)  [unwired: 7 in]
            "Last Error" <- w300
            n1216 = Match Pattern(string=w300, regular expression=w319) -> (match substring=w320:string)  [unwired: 1 in, 3 out]
            n1217 = Equal?(x=w320, y=w319) -> (x = y?=w299:bool)
            n1218 = Match Pattern(string=w300, regular expression=w301) -> (match substring=w302:string)  [unwired: 1 in, 3 out]
            n1219 = Equal?(x=w302, y=w301) -> (x = y?=w298:bool)
            n1220 = Or(x=w299, y=w298) -> (x .or. y?=w297:bool)
            n1221 = property on="Last Error" class="Str"(error in=w318, "Blinking"=w297) -> (error out=w303:errorcluster)  [unwired: 1 in, 1 out]
            n1222 = call "Read Instrument.lvclass.vi"("error in (no error)"=w303, "S4ACS_GUI in"=w305) -> ("error out"=w307:errorcluster, "Instrument.lvclass"=w306:refnum<class "Instrument.lvclass">, "S4ACS_GUI out"=w295:refnum<class "S4GUI.lvclass">)  [unwired: 7 in]
            n1223 = call-dynamic "Read mode.vi"("error in (no error)"=w307, "Instrument in"=w306) -> ("error out"=w296:errorcluster, "mode"=w308:bool)  [unwired: 7 in, 1 out]
            n1224 = while {
              tunnel: w308 -> [w351]
              shift-right: [w347] -> _
              shift-left: _ -> [w350]
              shift-right: [w348] -> _
              shift-left: _ -> [w349]
